vi "UE9 Logger Example.vi"() -> ()   [LabVIEW 2021]
panel:
  in  "ConnectionType":string="LJ_ctUSB"
  in  "AIN Range":u16(ring) items=["LJ_rgBIP5V", "LJ_rgUNI5V", "LJ_rgUNI2P5V", "LJ_rgUNI1P25V", "LJ_rgUNIP625V"]
  in  "FIO State":bool[](array[boolean])=[FALSE, FALSE, FALSE, FALSE, FALSE, FALSE, FALSE, FALSE]
  in  "FIO Direction (In=F,Out=T)":bool[](array[boolean])=[FALSE, FALSE, FALSE, FALSE, FALSE, FALSE, FALSE, FALSE]
  in  "DAC1":dbl format="%.4f"
  in  "DAC0":dbl format="%.4f"
  in  "Data File Extension":string="dat"
  out "Current Data File":path
  in  "Data File Prefix":string="data"
  in  "Write To File":bool
  in  "Update Interval (ms)":i32=500
  in  "FirstFound":bool=TRUE
  in  "stop":bool
  in  "Address":string="192.168.1.209"
  out "Reads":dbl[](array[numeric]) format="%.6f"
  out "Error Message":string
  in  "Resolution":i32=17
  # "AIN0"
  # "AIN1"
  # "AIN2"
  # "AIN3"
  # "AIN4"
  # "Specify an IP address for Ethernet, or Local ID\nfor USB.  If FirstFound is selected, Local ID is\nignored for USB.  Turn off FirstFound for Ethernet."
  # "AIN5"
  # "AIN6"
  # "(for all channels)"
  # "AIN7"
  # "AIN8"
  # "AIN9"
  # "AIN10"
  # "AIN11"
  # "0"
  # "1"
  # "2"
  # "3"
  # "4"
  # "5"
  # "6"
  # "7"
  # "AIN12"
  # "AIN13"
  # "Deg K"
  # "0"
  # "1"
  # "2"
  # "3"
  # "4"
  # "5"
  # "6"
  # "7"
  # "Vs"
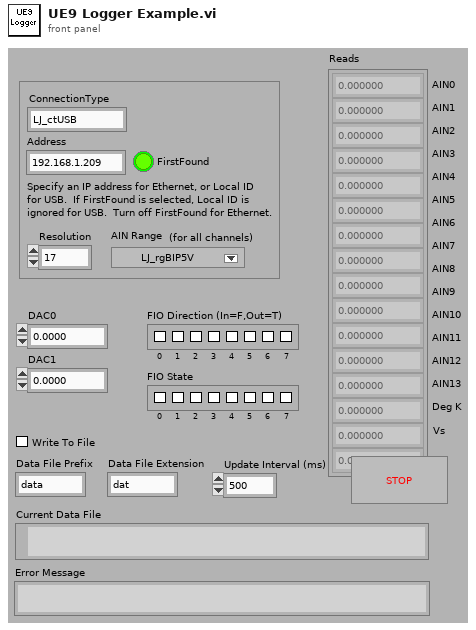
[diagram p1: front panel]
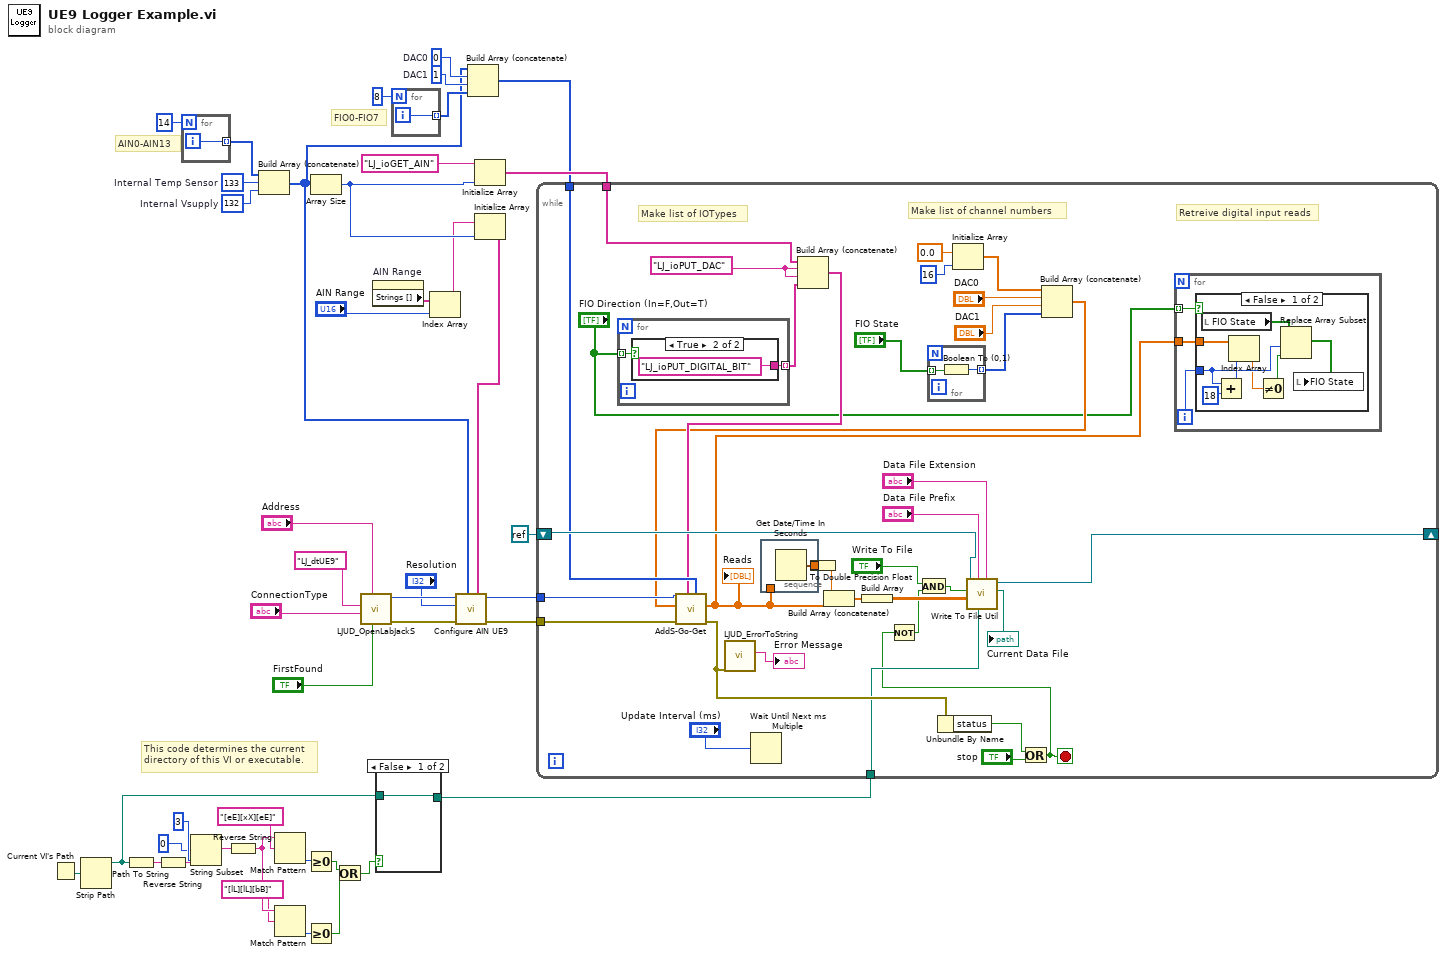
[diagram p0: block diagram]
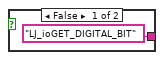
[diagram p3: hidden frame]
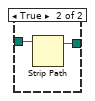
[diagram p4: hidden frame]
diagram:
  w9 = 1  # DAC1
  w10 = 0  # DAC0
  w15 = 132  # Internal Vsupply
  w14 = 133  # Internal Temp Sensor
  # "AIN0-AIN13"
  # "FIO0-FIO7"
  # "This code determines the current\ndirectory of this VI or executable."
  n1 = Current VI's Path() -> (path=w33:path)
  n2 = Strip Path(path=w33) -> (stripped path=w25:path)  [unwired: 1 out]
  n3 = Path To String(path=w25) -> (string=w32:string)
  n4 = Reverse String(1:w32) -> (0:w31:string)
  n5 = for {
    N: 14 -> [_]
    tunnel: [w44] -> w13 mode=indexing
    i -> [w44]
  }
  n6 = String Subset(string=w31, offset (0)=0, length (rest)=3 ("length")) -> (substring=w28:string)
  n7 = Reverse String(1:w28) -> (0:w24:string)
  n8 = Build Array (concatenate)(w13, w14, w15) -> (w8:i32[])
  n9 = Match Pattern(string=w24, regular expression="[eE][xX][eE]") -> (offset past match=w26:i32)  [unwired: 1 in, 3 out]
  n10 = Match Pattern(string=w24, regular expression="[lL][lL][bB]") -> (offset past match=w21:i32)  [unwired: 1 in, 3 out]
  n11 = Greater Or Equal To 0?(x=w26) -> (x >= 0?=w22:bool)
  n12 = Greater Or Equal To 0?(x=w21) -> (x >= 0?=w20:bool)
  n13 = Array Size(array=w8) -> (size(s)=w17:i32)
  n14 = Or(x=w22, y=w20) -> (x .or. y?=w19:bool)
  n15 = call "LJUD_OpenLabJackS.vi"("FirstFound"="FirstFound", "Address"="Address", "ConnectionType"="ConnectionType", "DeviceType"="LJ_dtUE9") -> ("error out"=w42:errorcluster, "Handle"=w43:i32)  [unwired: 5 in, 1 out]
  n16 = property on="AIN Range" class="Ring (strict)"() -> ("Strings []"=w6:string[])  [unwired: 2 in, 2 out]
  n17 = case shown="False" w19 {
    tunnel: w25 -> [w45 w47]
    tunnel: [w45 w46] -> w18
    frame False {
    }
    frame True {
      n18 = Strip Path(path=w47) -> (stripped path=w46:path)  [unwired: 1 out]
    }
  }
  n19 = for {
    N: 8 -> [_]
    tunnel: [w48] -> w11 mode=indexing
    i -> [w48]
  }
  n20 = Index Array(array=w6, index="AIN Range") -> (element=w4:string)
  n21 = Build Array (concatenate)(w8, w10, w9, w11) -> (w7:i32[])
  n22 = Initialize Array("LJ_ioGET_AIN" ("IOType"), w17) -> (w35:string[])
  n23 = Initialize Array(w4, w17) -> (w3:string[])
  n24 = call "Configure AIN UE9.vi"("Ranges"=w3, "Channels"=w8, "error in"=w42, "Resolution"="Resolution", "Handle In"=w43) -> ("error out"=w39:errorcluster, "Handle Out"=w40:i32)  [unwired: 5 in]
  n25 = while {
    tunnel: w7 -> [w62]
    tunnel: w18 -> [w67]
    shift-left: refnum<k0> refnum -> [w74]
    shift-right: [w73] -> _
    tunnel: w35 -> [w61]
    tunnel: w39 -> [w82]
    tunnel: w40 -> [w66]
    stop <- w64 stop-if-true
    w49 = "LJ_ioPUT_DAC" ("IOType")
    # "Retreive digital input reads"
    # "Make list of channel numbers"
    # "Make list of IOTypes"
    n26 = for {
      tunnel: "FIO Direction (In=F,Out=T)" -> [w98] mode=indexing
      tunnel: [w97] -> w63 mode=indexing
      n27 = case shown="True" w98 {
        tunnel: ["LJ_ioGET_DIGITAL_BIT" ("IOType") "LJ_ioPUT_DIGITAL_BIT" ("IOType")] -> w97
        frame False {
        }
        frame True {
        }
      }
    }
    n28 = Wait Until Next ms Multiple(millisecond multiple="Update Interval (ms)") -> ()  [unwired: 1 out]
    n29 = Build Array (concatenate)(w61, w49, w49, w63) -> (w60:string[])
    n30 = for {
      tunnel: "FIO State" -> [w96] mode=indexing
      tunnel: [w95] -> w59 mode=indexing
      n31 = Boolean To (0,1)(Boolean=w96) -> (0, 1=w95:i16)
    }
    n32 = Initialize Array(0.0 ("Element Data"), 16 ("Dimension Size")) -> (w56:dbl[])
    n33 = Build Array (concatenate)(w56, "DAC0", "DAC1", w59) -> (w52:dbl[])
    n34 = call "AddS-Go-Get.vi"("Channels"=w62, "IOTypes"=w60, "error in"=w82, "Values Write"=w52, "Handle In"=w66) -> ("error out"=w71:errorcluster, "Values Read"=w50:dbl[])  [unwired: 4 in, 1 out]
    "Reads" <- w50
    n35 = call "LJUD_ErrorToString.vi"("error in"=w71) -> ("String"=→"Error Message":string)  [unwired: 10 in]
    n36 = stacked-sequence {
      tunnel: [w102] -> w65
      tunnel: w50 -> [_]
      frame #0 {
        n37 = Get Date/Time In Seconds() -> (seconds since 1Jan1904=w101:timestamp)
        n38 = To Double Precision Float(number=w101) -> (double precision float=w102:dbl)
      }
    }
    n39 = Build Array (concatenate)(w65, w50) -> (w78:dbl[])
    n40 = Build Array(w78) -> (w77:dbl[][])
    n41 = Unbundle By Name(w71) -> ("status"=w80:bool)
    n42 = Or(x=w80, y="stop") -> (x .or. y?=w64:bool)
    n43 = Not(x=w64) -> (.not. x?=w68:bool)
    n44 = And(x="Write To File", y=w68) -> (x .and. y?=w69:bool)
    n45 = call "Write To File Util.vi"("Data File Extension"="Data File Extension", "Working Directory"=w67, "Data File Prefix"="Data File Prefix", "Data"=w77, "Write To File"=w69, "File Refnum In"=w74) -> ("Current Data File"=→"Current Data File":path, "File Refnum Out"=w73:refnum<file>)  [unwired: 3 in, 1 out]
    n46 = for {
      tunnel: "FIO Direction (In=F,Out=T)" -> [w86] mode=indexing
      tunnel: w50 -> [w84]
      i -> [w85]
      n47 = case shown="False" w86 {
        tunnel: w85 -> [w90 _]
        tunnel: w84 -> [w92 _]
        frame False {
          n48 = local read "FIO State"() -> (w91:bool[])
          n49 = Add(x=w90, y=18) -> (x+y=w93:i32)
          n50 = Index Array(array=w92, index=w93) -> (element=w88:dbl)
          n51 = Not Equal To 0?(x=w88) -> (x != 0?=w87:bool)
          n52 = Replace Array Subset(array=w91, new element=w87, index=w90) -> (w89:bool[])
          n53 = local write "FIO State"(w89) -> ()
        }
        frame True {
        }
      }
    }
  }
